vi "E7_Cluster1.vi"() -> ()   [LabVIEW 2020]
panel:
  out "output cluster 3":cluster{i32, dbl, bool, string}
  out "output cluster 2":T1
  out "output cluster":T2
  in  "Cluster":T1 {"Slide" scale=0.0..10.0}
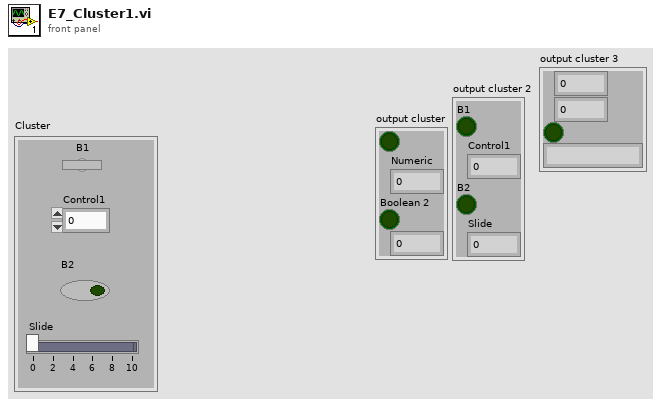
[diagram p1: front panel]
types:
  T1 = cluster{"B1":bool, "Control1":dbl, "B2":bool, "Slide":dbl}
  T2 = cluster{bool, "Numeric":dbl, "Boolean 2":bool, dbl}
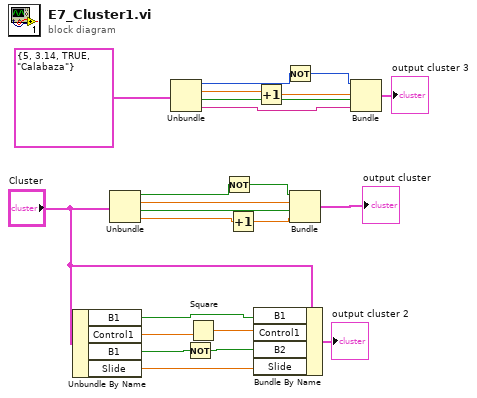
[diagram p0: block diagram]
diagram:
  n1 = Unbundle By Name "Unbundle By Name"("Cluster") -> ("B1"=w16:bool, "Control1"=w15:dbl, "B1"=w13:bool, "Slide"=w11:dbl)
  n2 = Unbundle "Unbundle"("Cluster") -> ("B1"=w22:bool, "Control1"=w19:dbl, "B2"=w18:bool, "Slide"=w23:dbl)
  n3 = Unbundle "Unbundle"(cluster{i32, dbl, bool, string} {5, 3.14, TRUE, "Calabaza"}) -> (w8:i32, w4:dbl, w6:bool, w2:string)
  n4 = Not(x=w13) -> (.not. x?=w12:bool)
  n5 = Square(x=w15) -> (x^2=w14:dbl)
  n6 = Not(x=w22) -> (.not. x?=w21:bool)
  n7 = Increment(x=w23) -> (x+1=w20:dbl)
  n8 = Bundle By Name "Bundle By Name"(cluster="Cluster", "B1"=w16, "Control1"=w14, "B2"=w12, "Slide"=w11) -> (→"output cluster 2":T1)
  n9 = Increment(x=w4) -> (x+1=w3:dbl)
  n10 = Not(x=w8) -> (.not. x?=w7:i32)
  n11 = Bundle "Bundle"(w21, "Control1"=w19, "B2"=w18, w20) -> (→"output cluster":cluster{bool, "Control1":dbl, "B2":bool, dbl})  [unwired: 1 in]
  n12 = Bundle "Bundle"(w7, w3, w6, w2) -> (→"output cluster 3":cluster{i32, dbl, bool, string})  [unwired: 1 in]
